vi "Agilent E363X Series Output DC Volts - Triggered.vi"() -> ()   [LabVIEW 2015]
doc: "This example demonstrates the triggering functionality of the power supply. Initial and triggered voltage and limit settings are configured. The Send Software Trigger VI is used to trigger the instrument."
uses:
  Agilent E363X Series.lvlib
panel:
  in  "Triggered Current Limit (1.0 A)":dbl=1.0 format="%.2g"
  in  "Current Limit (1.0 A)":dbl=1.0 format="%.3g"
  out "Post-trigger Voltage Level (V)":dbl format="%.3g"
  out "Post-trigger Current Level (A)":dbl format="%.3g"
  in  "Triggered Voltage Level (5.0 V)":dbl=5.0 format="%.3g"
  in  "Voltage Level (1.0 V)":dbl=1.0 format="%.3g"
  out "Pre-trigger Voltage Level (V)":dbl format="%.3g"
  out "Pre-trigger Current Level (A)":dbl format="%.3g"
  in  "VISA resource name":refnum<visa-resource-name>
  # "(c) 2008 National Instruments.  ALL RIGHTS RESERVED."
  # "Initial Voltage Settings"
  # "Triggered Settings"
  # "Post-trigger Levels"
  # "Pre-trigger Levels"
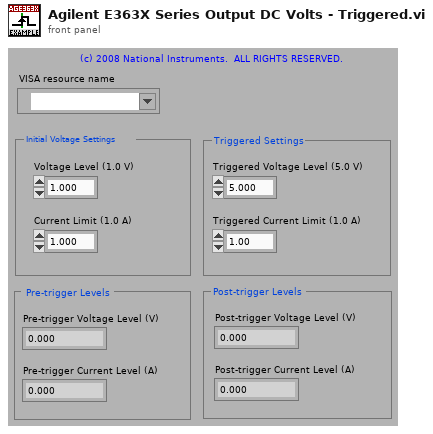
[diagram p1: front panel]
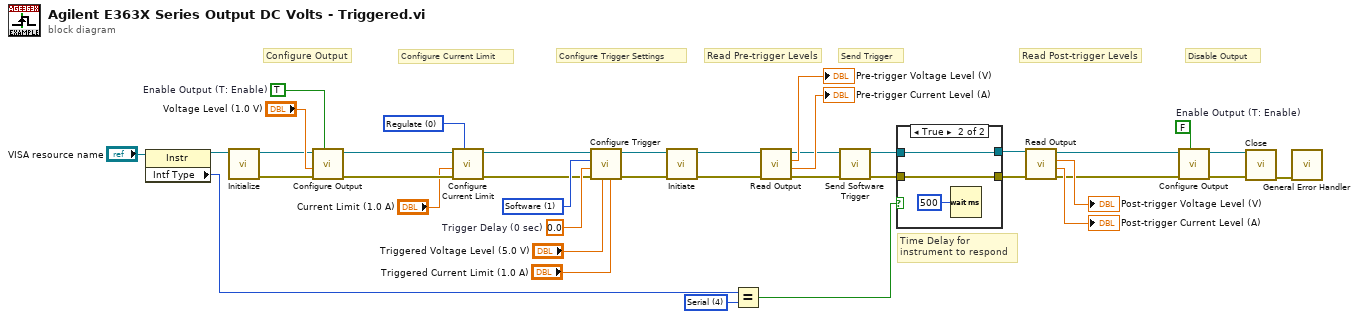
[diagram p0: block diagram]
diagram:
  w2 = u16 4 items=["GPIB"=1, "VXI"=2, "GPIB-VXI"=3, "Serial"=4, "PXI"=5, "TCPIP"=6, "USB"=7] ("Interface Information:Interface Type")
  w12 = u16 0 items=["Regulate", "Trip"] ("Behavior (0: Regulate)")
  w30 = 0.0  # Trigger Delay (0 sec)
  w31 = u16 1 items=["Immediate", "Software"] ("Trigger Source (0: Immediate)")
  w35 = TRUE  # Enable Output (T: Enable)
  w38 = FALSE  # Enable Output (T: Enable)
  # "Time Delay for instrument to respond"
  # "Configure Current Limit"
  # "Read Post-trigger Levels"
  # "Read Pre-trigger Levels"
  # "Disable Output"
  # "Send Trigger"
  # "Configure Trigger Settings"
  # "Configure Output"
  n1 = property class="Instr"(reference="VISA resource name") -> (reference out=w5:refnum<visa-resource-name>, "Intf Type"=w3:u16)  [unwired: 1 in, 1 out]
  n2 = call "Initialize.vi"("VISA resource name"=w5) -> ("error out"=w25:errorcluster, "VISA resource name out"=w26:refnum<visa-resource-name>)  [unwired: 9 in]
  n3 = call "Configure Output.vi"("Enable Output (T: Enable)"=w35, "error in (no error)"=w25, "Voltage Level (0.0 V)"="Voltage Level (1.0 V)", "VISA resource name"=w26) -> ("error out"=w15:errorcluster, "VISA resource name out"=w16:refnum<visa-resource-name>)  [unwired: 6 in]
  n4 = call "Configure Current Limit.vi"("Behavior (0: Regulate)"=w12, "error in (no error)"=w15, "Current Limit (0.0 A)"="Current Limit (1.0 A)", "VISA resource name"=w16) -> ("error out"=w13:errorcluster, "VISA resource name out"=w14:refnum<visa-resource-name>)  [unwired: 6 in]
  n5 = call "Configure Trigger.vi"("Triggered Current Limit (0.0 A)"="Triggered Current Limit (1.0 A)", "Triggered Voltage Level (0.0 V)"="Triggered Voltage Level (5.0 V)", "error in (no error)"=w13, "Trigger Delay (0 sec)"=w30, "Trigger Source (0: Immediate)"=w31, "VISA resource name"=w14) -> ("error out"=w32:errorcluster, "VISA resource name out"=w33:refnum<visa-resource-name>)  [unwired: 4 in]
  n6 = call "Initiate.vi"("error in (no error)"=w32, "VISA resource name"=w33) -> ("error out"=w27:errorcluster, "VISA resource name out"=w28:refnum<visa-resource-name>)  [unwired: 8 in]
  n7 = Equal?(x=w3, y=w2) -> (x = y?=w1:bool)
  n8 = call "Read Output.vi"("error in (no error)"=w27, "VISA resource name"=w28) -> ("error out"=w21:errorcluster, "Actual Current Level (A)"=→"Pre-trigger Current Level (A)":dbl, "Actual Voltage Level (V)"=→"Pre-trigger Voltage Level (V)":dbl, "VISA resource name out"=w22:refnum<visa-resource-name>)  [unwired: 6 in]
  n9 = call "Send Software Trigger.vi"("error in (no error)"=w21, "VISA resource name"=w22) -> ("error out"=w7:errorcluster, "VISA resource name out"=w9:refnum<visa-resource-name>)  [unwired: 8 in]
  n10 = case shown="True" w1 {
    tunnel: [w41 w43] -> w8
    tunnel: w9 -> [w41 w43]
    tunnel: [w40 w42] -> w6
    tunnel: w7 -> [w40 w42]
    frame False {
    }
    frame True {
      n11 = Wait (ms)(milliseconds to wait=u32 500) -> ()  [unwired: 1 out]
    }
  }
  n12 = call "Read Output.vi"("error in (no error)"=w6, "VISA resource name"=w8) -> ("error out"=w18:errorcluster, "Actual Current Level (A)"=→"Post-trigger Current Level (A)":dbl, "Actual Voltage Level (V)"=→"Post-trigger Voltage Level (V)":dbl, "VISA resource name out"=w17:refnum<visa-resource-name>)  [unwired: 6 in]
  n13 = call "Configure Output.vi"("Enable Output (T: Enable)"=w38, "error in (no error)"=w18, "VISA resource name"=w17) -> ("error out"=w36:errorcluster, "VISA resource name out"=w37:refnum<visa-resource-name>)  [unwired: 7 in]
  n14 = call "Close.vi"("error in (no error)"=w36, "VISA resource name"=w37) -> ("error out"=w39:errorcluster)  [unwired: 9 in]
  n15 = call <vilib>:"General Error Handler.vi"("error in (no error)"=w39) -> ()  [unwired: 10 in, 5 out]
